vi "all-signals+drivingtorque.vi"() -> ()   [LabVIEW 2018]
panel:
  in  "Clear Charts":bool
  in  "stop clear charts":bool
  in  "stop  counter (F)":bool caption="counter stop (F)"
  in  "stop I,U,M_brems (F)":bool caption="IU P STOP (F)"
  out "Driving Torque":dynamicdata(graph)
  out "RPM":dbl
  in  "Messzeit in ms":u32=100 min=10 max=1000 step=10
  out "Bremsmoment":dynamicdata(graph)
  out "Strom, Spannung, elektrische Leistung":dynamicdata(graph)
  out "Geschwindigkeit":dynamicdata(graph)
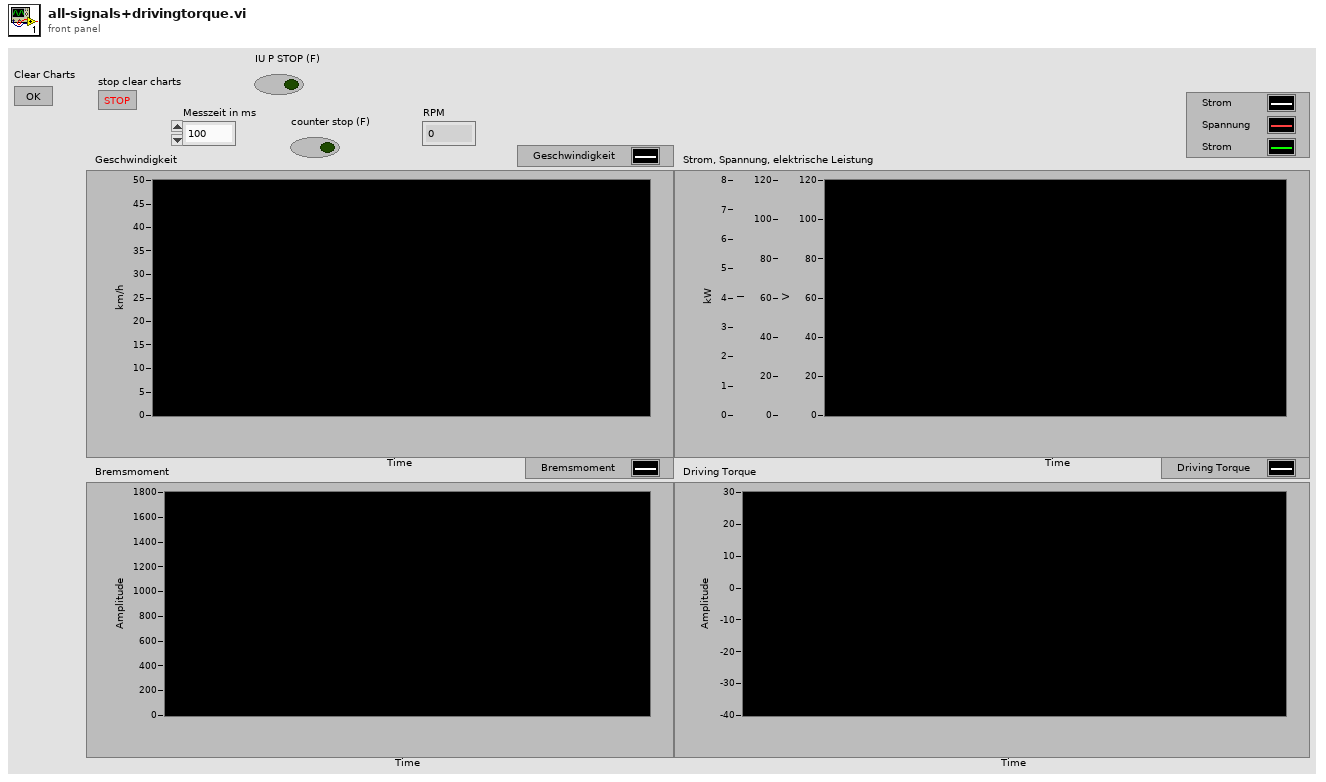
[diagram p1: front panel]
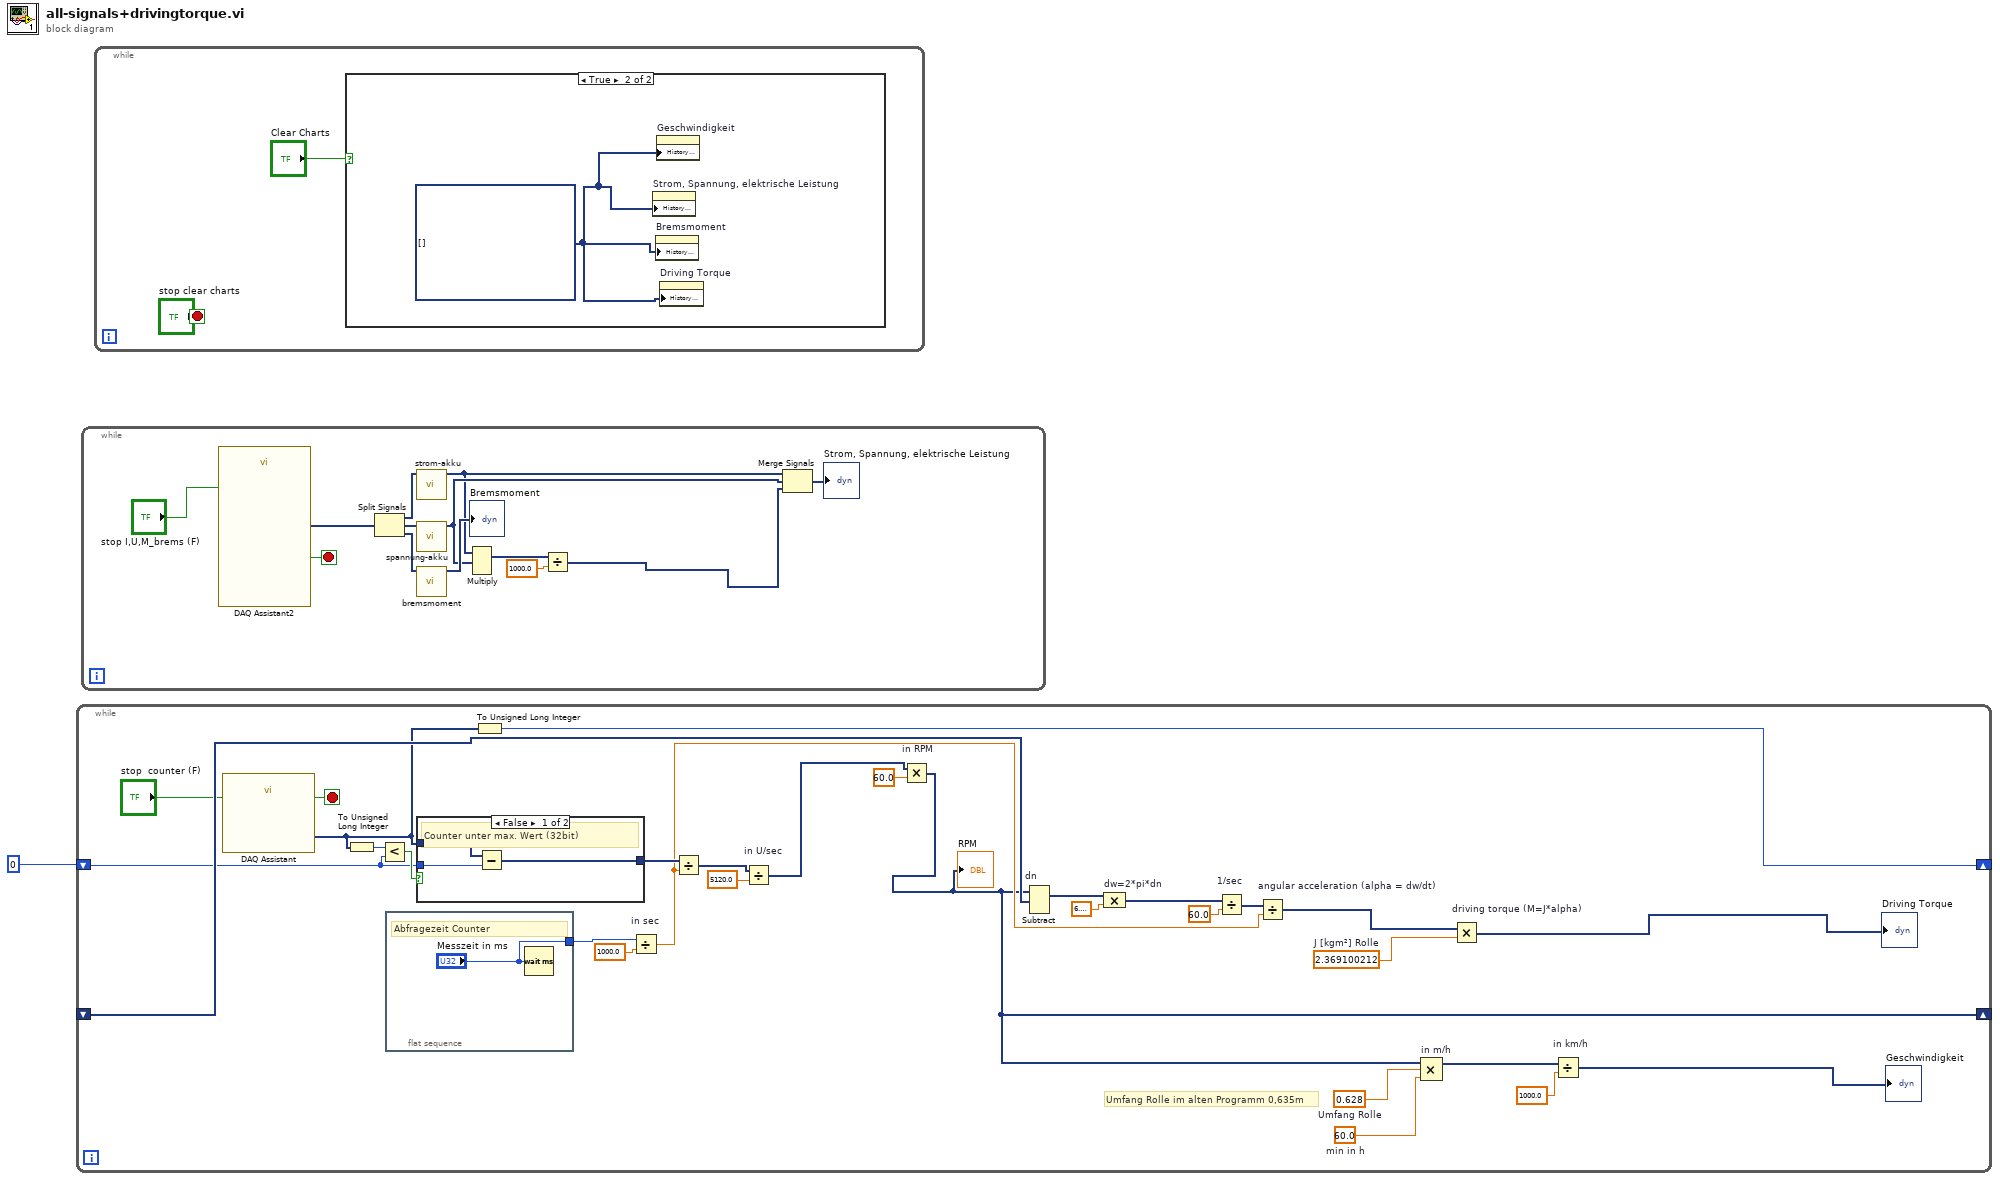
[diagram p0: block diagram]
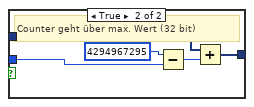
[diagram p2: hidden frame]
diagram:
  n1 = while {
    shift-right: [w29] -> _
    shift-left: u32 0 -> [w3]
    shift-right: [w2] -> _
    shift-left: _ -> [w20]
    stop <- w27 stop-if-true
    w12 = 2.369100212  # J [kgm²] Rolle
    w10 = 60.0  # min in h
    w9 = 0.628  # Umfang Rolle
    # "Umfang Rolle im alten Programm 0,635m"
    n2 = call "DAQ Assistant"("stop (F)"="stop  counter (F)") -> ("data"=w4:dynamicdata, "stopped"=w27:bool)  [unwired: 15 in, 2 out]
    n3 = To Unsigned Long Integer(number=w4) -> (unsigned 32bit integer=w28:u32)
    n4 = Less?(x=w28, y=w3) -> (x < y?=w31:bool)
    n5 = flat-sequence {
      tunnel: ["Messzeit in ms"] -> w26
      frame #0 {
        # "Abfragezeit Counter"
        n6 = Wait (ms)(milliseconds to wait="Messzeit in ms") -> ()  [unwired: 1 out]
      }
    }
    n7 = case shown="False" w31 {
      tunnel: w4 -> [w35 w37]
      tunnel: w3 -> [w34 w39]
      tunnel: [w33 w36] -> w24
      frame False {
        # "Counter unter max. Wert (32bit)"
        n8 = Subtract(x=w35, y=w34) -> (x-y=w33:dynamicdata)
      }
      frame True {
        # "Counter geht über max. Wert (32 bit)"
        n9 = Subtract(x=u32 4294967295, y=w39) -> (x-y=w38:u32)
        n10 = Add(x=w37, y=w38) -> (x+y=w36:dynamicdata)
      }
    }
    n11 = To Unsigned Long Integer(number=w4) -> (unsigned 32bit integer=w29:u32)
    n12 = Divide "in sec"(x=w26, y=1000.0) -> (x/y=w15:dbl)
    n13 = Divide(x=w24, y=w15) -> (x/y=w23:dynamicdata)
    n14 = Divide "in U/sec"(x=w23, y=5120.0) -> (x/y=w7:dynamicdata)
    n15 = Multiply "in RPM"(x=w7, y=60.0) -> (x*y=w2:dynamicdata)
    "RPM" <- w2
    n16 = Subtract "dn"(1:w20, 2:w2) -> (0:w19:dynamicdata)  [unwired: 1 in, 1 out]
    n17 = Compound Arithmetic op=MULTIPLY "dw=2*pi*dn"(w19, 6.283185307179586) -> (w18:dynamicdata)
    n18 = Divide "1/sec"(x=w18, y=60.0) -> (x/y=w16:dynamicdata)
    n19 = Divide "angular acceleration (alpha = dw/dt)"(x=w16, y=w15) -> (x/y=w13:dynamicdata)
    n20 = Compound Arithmetic op=MULTIPLY "in m/h"(w2, w9, w10) -> (w11:dynamicdata)
    n21 = Multiply "driving torque (M=J*alpha)"(x=w13, y=w12) -> (x*y=→"Driving Torque":dynamicdata)
    n22 = Divide "in km/h"(x=w11, y=1000.0) -> (x/y=→"Geschwindigkeit":dynamicdata)
  }
  n23 = while {
    stop <- w47 stop-if-true
    n24 = call "DAQ Assistant2"("stop (F)"="stop I,U,M_brems (F)") -> ("data"=w48:dynamicdata, "stopped"=w47:bool)  [unwired: 15 in, 2 out]
    n25 = Split Signals(w48) -> (w53:dynamicdata, w52:dynamicdata, w51:dynamicdata)  [unwired: 3 in]
    n26 = call "strom-akku.vi"("Dynamic Data"=w53) -> ("Filtered Signal"=w45:dynamicdata)  [unwired: 10 in]
    n27 = call "spannung-akku.vi"("Dynamic Data in"=w52) -> ("Dynamic Data out"=w46:dynamicdata)  [unwired: 10 in]
    n28 = call "bremsmoment.vi"("Dynamic Data in"=w51) -> ("Dynamic Data out"=→"Bremsmoment":dynamicdata)  [unwired: 10 in]
    n29 = Multiply(1:w46, 2:w45) -> (0:w43:dynamicdata)  [unwired: 1 in, 1 out]
    n30 = Divide(x=w43, y=1000.0) -> (x/y=w41:dynamicdata)
    n31 = Merge Signals(w45, w46, w41) -> (→"Strom, Spannung, elektrische Leistung":dynamicdata)
  }
  n32 = while {
    stop <- "stop clear charts" stop-if-true
    n33 = case shown="True" "Clear Charts" {
      frame False {
      }
      frame True {
        w56 = dynamicdata[] [] ("History Data")
        n34 = property on="Strom, Spannung, elektrische Leistung" class="WFChart (strict)"("History Data"=w56) -> ()  [unwired: 2 in, 2 out]
        n35 = property on="Bremsmoment" class="WFChart (strict)"("History Data"=w56) -> ()  [unwired: 2 in, 2 out]
        n36 = property on="Geschwindigkeit" class="WFChart (strict)"("History Data"=w56) -> ()  [unwired: 2 in, 2 out]
        n37 = property on="Driving Torque" class="WFChart (strict)"("History Data"=w56) -> ()  [unwired: 2 in, 2 out]
      }
    }
  }
